vi "Camera software flag.vi"() -> ()   [LabVIEW 2020]
panel:
  in  "Camera software flag":dbl
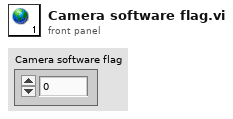
[diagram p1: front panel]
diagram:
